vi "Untitled 15.vi"() -> ()   [LabVIEW 2010]
uses:
  countdown control.ctl
panel:
  in  "timer \"v\"":dbl(slide)=0.29032258064516125 min=-1725004073.0 max=1.0 step=0.01 scale=0.0..50.0 scale format="%#_2g"
  in  "timer \"o\"":dbl(slide)=0.29032258064516125 min=-1725003981.0 max=1.0 step=0.01 scale=0.0..80.0 scale format="%#_2g"
  in  "autopilot":bool
  in  "\"v\" interval (sec)":dbl=70.0
  in  "\"o\" interval (sec)":dbl=90.0
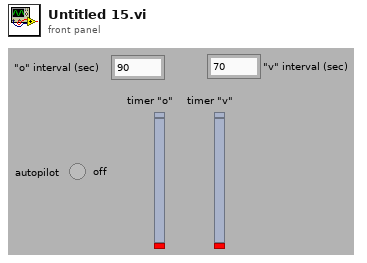
[diagram p1: front panel]
types:
  T1 = typedef "countdown control.ctl" = enum16{"check", "start", "reset"}
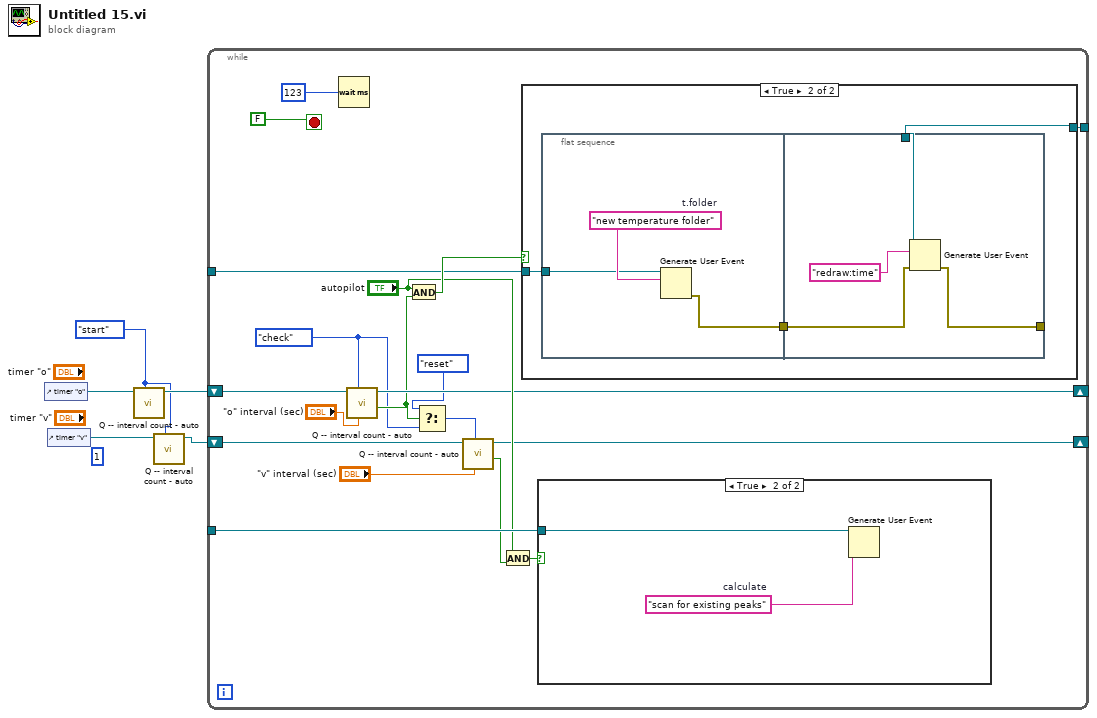
[diagram p0: block diagram]
diagram:
  w1 = countdown_control."start" ("action")
  (unwired) 1
  n1 = control-ref of="timer \"o\""() -> (w5:refnum<vi>)
  n2 = control-ref of="timer \"v\""() -> (w4:refnum<vi>)
  n3 = call "Q -- interval count - auto.vi"("action"=w1, "timer in"=w5) -> ("timer out"=w3:refnum<vi>)  [unwired: 7 in, 2 out]
  n4 = call "Q -- interval count - auto.vi"("action"=w1, "timer in"=w4) -> ("timer out"=w2:refnum<vi>)  [unwired: 7 in, 2 out]
  n5 = while {
    tunnel: [w23] -> w7
    tunnel: _ -> [w22]
    tunnel: [w20] -> w6
    shift-right: [w17] -> _
    shift-left: w3 -> [w18]
    shift-right: [w13] -> _
    shift-left: w2 -> [w16]
    stop <- FALSE stop-if-true
    w9 = countdown_control."check" ("action")
    n6 = Wait (ms)(milliseconds to wait=u32 123) -> ()  [unwired: 1 out]
    n7 = call "Q -- interval count - auto.vi"("interval (sec)"="\"o\" interval (sec)", "action"=w9, "timer in"=w18) -> ("tic"=w11:bool, "timer out"=w17:refnum<vi>)  [unwired: 6 in, 1 out]
    n8 = And(x="autopilot", y=w11) -> (x .and. y?=w24:bool)
    n9 = Select(t=countdown_control."reset" ("action"), s=w11, f=w9) -> (s? t:f=w8:T1)
    n10 = call "Q -- interval count - auto.vi"("interval (sec)"="\"v\" interval (sec)", "action"=w8, "timer in"=w16) -> ("tic"=w12:bool, "timer out"=w13:refnum<vi>)  [unwired: 6 in, 1 out]
    n11 = And(x="autopilot", y=w12) -> (x .and. y?=w21:bool)
    n12 = case shown="True" w24 {
      tunnel: w23 -> [_ w30]
      tunnel: w22 -> [_ w29]
      frame False {
      }
      frame True {
        n13 = flat-sequence {
          tunnel: w30 -> [w33]
          tunnel: [w32] -> w31
          tunnel: [w35] -> _
          tunnel: w31 -> [w36]
          tunnel: w29 -> [w37]
          frame #0 {
            w34 = "new temperature folder"  # t.folder
            n14 = Generate User Event(user event=w33, event data cluster=w34) -> (error out=w32:errorcluster)  [unwired: 1 in, 1 out]
          }
          frame #1 {
            n15 = Generate User Event(user event=w37, event data cluster="redraw:time", error in=w36) -> (error out=w35:errorcluster)  [unwired: 1 out]
          }
        }
      }
    }
    n16 = case shown="True" w21 {
      tunnel: w20 -> [_ w27]
      frame False {
      }
      frame True {
        w28 = "scan for existing peaks"  # calculate
        n17 = Generate User Event(user event=w27, event data cluster=w28) -> ()  [unwired: 1 in, 2 out]
      }
    }
  }
